vi "Configure Timebase.vi"(8 "error in (no error)":errorcluster, 9 "Offset (0.0 s)":dbl, 10 "Timebase (0.0005 s)":dbl=0.0005, 11 "VISA resource name":refnum<visa-resource-name>) -> (0 "error out":errorcluster, 3 "VISA resource name out":refnum<visa-resource-name>)   [LabVIEW 2015, in "RIGOL DS1000 Series.lvlib"]
doc: "Configures the timebase and horizontal features of the oscilloscope."
uses:
  RIGOL DS1000 Series.lvlib
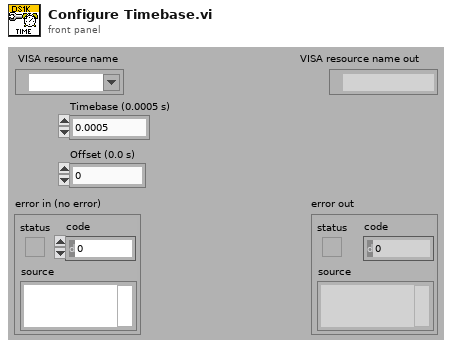
[diagram p1: front panel]
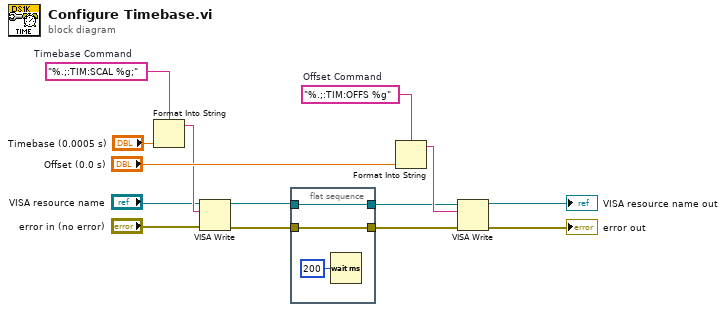
[diagram p0: block diagram]
diagram:
  w10 = "%.;:TIM:OFFS %g"  # Offset Command
  w11 = "%.;:TIM:SCAL %g;"  # Timebase Command
  n1 = Format Into String(format string=w11, "Timebase (0.0005 s)") -> (resulting string=w8:string)  [unwired: 2 in, 1 out]
  n2 = VISA Write(VISA resource name="VISA resource name", write buffer=w8, error in (no error)="error in (no error)") -> (VISA resource name out=w3:refnum<visa-resource-name>, error out=w4:errorcluster)  [unwired: 1 out]
  n3 = flat-sequence {
    tunnel: [w16] -> w6
    tunnel: w3 -> [w16]
    tunnel: w4 -> [w15]
    tunnel: [w15] -> w5
    frame #0 {
      n4 = Wait (ms)(milliseconds to wait=u32 200) -> ()  [unwired: 1 out]
    }
  }
  n5 = Format Into String(format string=w10, "Offset (0.0 s)") -> (resulting string=w12:string)  [unwired: 2 in, 1 out]
  n6 = VISA Write(VISA resource name=w6, write buffer=w12, error in (no error)=w5) -> (VISA resource name out=→"VISA resource name out":refnum<visa-resource-name>, error out=→"error out":errorcluster)  [unwired: 1 out]
